vi "Reset Wifi.vi"(7 "Retry wait time [ms]":u32=100, 8 "error in (no error)":errorcluster, 11 "LINX Resource":T1) -> (0 "error out":errorcluster, 1 "Connected to network?":bool, 2 "TCP Config":T5, 3 "LINX Resource Out":T1)   [LabVIEW 2019, in "LINXx.lvlib"]
doc: "Resets board's WiFi connection"
uses:
  LINXx.lvlib
  <vilib>/MakerHub/LINX/Private/Type Defs/LINX Ref.ctl
  <vilib>/MakerHub/LINX/Private/Type Defs/Platform.ctl
  <vilib>/MakerHub/LINX/Private/Type Defs/Interface.ctl
  <vilib>/MakerHub/LINX/Private/Device/Type Defs/LINX Device Config.ctl
  <vilib>/MakerHub/LINX/Private/Device/Type Defs/TCP Config.ctl
  <vilib>/MakerHub/LINX/Private/Device/Type Defs/Channels.ctl
  Public/Reset Target.ctl
  WiFi101 Status.ctl
  <vilib>/MakerHub/LINX/LMH-LINX.lvlib
  <vilib>/MakerHub/LINX/Private/Device/Device.lvlib
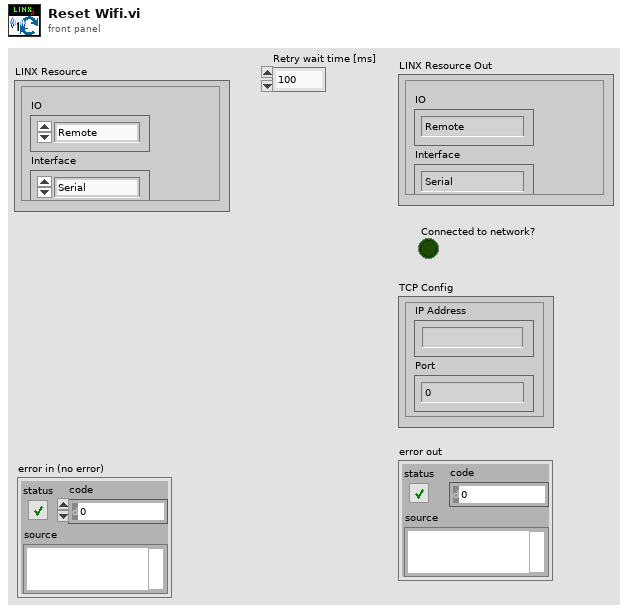
[diagram p1: front panel]
types:
  T1 = typedef "LMH-LINX.lvlib/LINX Ref.ctl" = cluster{"IO":T2, "Interface":T3, "LINX Device Config":T4}
  T2 = typedef "LMH-LINX.lvlib/Platform.ctl" = enum16{"Remote", "Local"}
  T3 = typedef "LMH-LINX.lvlib/Interface.ctl" = enum16{"Serial", "TCP"}
  T4 = typedef "LMH-LINX.lvlib/Device.lvlib/LINX Device Config.ctl" = cluster{"Interface":T3, "COM Port":refnum<visa-resource-name>, "TCP Configuration":T5, "Device Family":u8, "Device ID":u8, "Device Name":string, "TCP Ref":refnum<k5>, "Channels":T6}
  T5 = typedef "LMH-LINX.lvlib/Device.lvlib/TCP Config.ctl" = cluster{"IP Address":string, "Port":u16}
  T6 = typedef "LMH-LINX.lvlib/Channels.ctl" = cluster{"DI":u8[], "DO":u8[], "AI":u8[], "AO":u8[], "PWM":u8[], "QE":u8[], "UART":u8[], "I2C 2":u8[], "SPI":u8[], "CAN":u8[], "Servo":u8[], "AI Ref (V)":dbl, "AI Resolution (Bits)":u8, "AO Ref (V)":dbl, "AO Resolution (Bits)":u8}
  T7 = typedef "LINXx.lvlib/WiFi101 Status.ctl" = u8
  T8 = typedef "LINXx.lvlib/Reset Target.ctl" = enum16{"None", "Serial", "TCP", "Board"}
  T9 = typedef "LMH-LINX.lvlib/Device.lvlib/Wifi Config.ctl" = cluster{"SSID":string, "IP Address":string, "Port":u16, "WIFI Security Type":T10, "Password":string}
  T10 = typedef "LMH-LINX.lvlib/WIFI Security Type.ctl" = enum8{"None", "WPA2 Password", "WPA2 Key", "WEP40", "WEP104"}
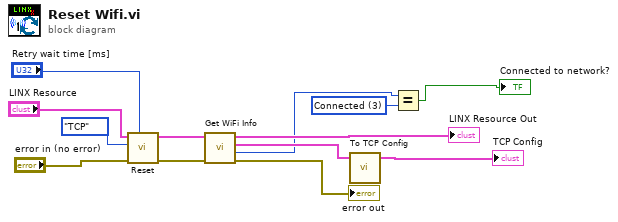
[diagram p0: block diagram]
diagram:
  w2 = T7 3 items=["No module"=255, "Idle"=0, "No SSID"=1, "Scan completed"=2, "Connected"=3, "Connection failed"=4, "Connection lost"=5, "Disconnected"=6, "AP listening"=7, "AP connected"=8, "AP failed"=9, "Provisioning"=10, "Provisioning failed"=11] ("Ring")
  n1 = call "Reset.vi"("Reconnect \nwait time [ms]"="Retry wait time [ms]", "Error In"="error in (no error)", "Reset Target"=Reset_Target."TCP" ("f"), "LINX Resource"="LINX Resource") -> ("Error Out"=w11:errorcluster, "LINX Resource out"=w10:T1)  [unwired: 6 in]
  n2 = call "Get WiFi Info.vi"("Error In"=w11, "LINX Resource"=w10) -> ("Error Out"=→"error out":errorcluster, "WiFi status"=w1:u8, "WiFi Info"=w5:T9, "LINX Resource Out"=→"LINX Resource Out":T1)  [unwired: 6 in]
  n3 = call "To TCP Config.vi"("Wifi Configuration"=w5) -> ("TCP Configuration"=→"TCP Config":T5)  [unwired: 4 in]
  n4 = Equal?(x=w1, y=w2) -> (x = y?=→"Connected to network?":bool)
